vi "Utility Save Restore Setup.vi"(0 "VISA resource name":refnum<visa-resource-name>, 2 "Operation (0: Restore)":u16(ring) items=["Restore", "Save"], 5 "error in (no error)":errorcluster) -> (14 "VISA resource name out":refnum<visa-resource-name>, 19 "error out":errorcluster)   [LabVIEW 2009, in "Keithley 2000.lvlib"]
doc: "This VI restores previously saved configuration information on the instrument or saves the current configuration information to be restored later."
uses:
  <instrlib>/Keithley 2000/Keithley 2000.lvlib
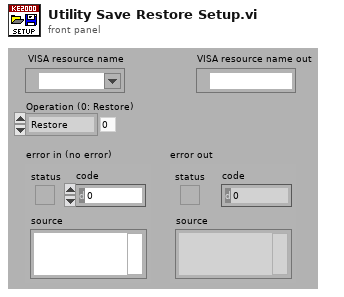
[diagram p1: front panel]
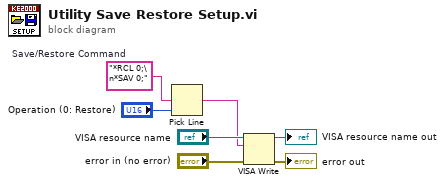
[diagram p0: block diagram]
diagram:
  w3 = "*RCL 0;\n*SAV 0;"  # Save/Restore Command
  n1 = Pick Line(multi-line string=w3, line index="Operation (0: Restore)") -> (output string=w1:string)  [unwired: 1 in]
  n2 = VISA Write(VISA resource name="VISA resource name", write buffer=w1, error in (no error)="error in (no error)") -> (VISA resource name out=→"VISA resource name out":refnum<visa-resource-name>, error out=→"error out":errorcluster)  [unwired: 1 out]
